vi "Close Device.vi"(8 "error in (no error)":errorcluster, 11 "Device in":refnum<class "Toggle 8.lvclass">) -> (0 "error out":errorcluster, 3 "Device out":refnum<class "Toggle 8.lvclass">)   [LabVIEW 2020, in "Toggle 8.lvclass"]
doc: "Closes the device"
uses:
  Toggle 8.lvclass
  PIC-device/PIC-Device.lvclass
  <instrlib>/Keithley 24XX/Keithley 24XX.lvlib
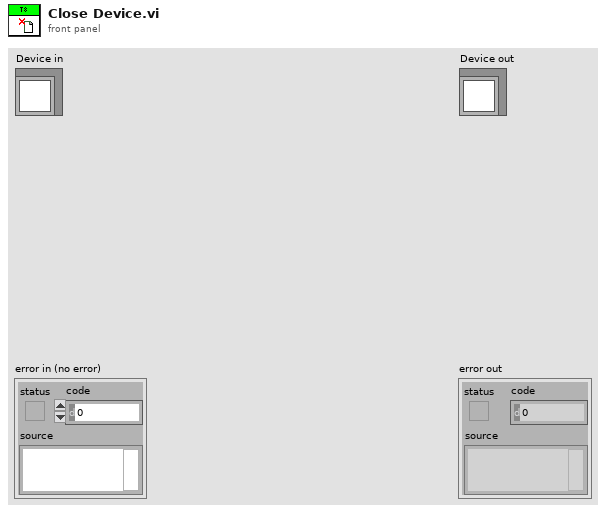
[diagram p1: front panel]
types:
  T1 = cluster{"Enable":bool, "User init values":string}
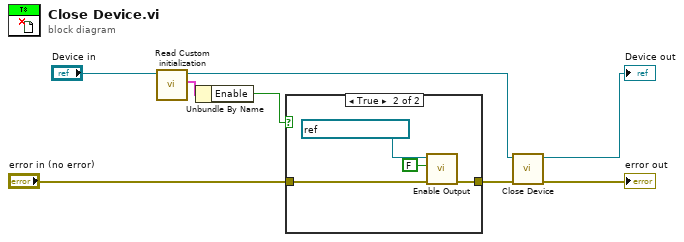
[diagram p0: block diagram]
diagram:
  n1 = call-dynamic "Read Custom initialization.vi"("Toggle 8 in"="Device in") -> ("Custom initialization"=w4:T1, "Toggle 8 out"=w5:refnum<class "Toggle 8.lvclass">)  [unwired: 9 in]
  n2 = Unbundle By Name(w4) -> ("Enable"=w1:bool)
  n3 = case shown="True" w1 {
    tunnel: "error in (no error)" -> [w9 w12]
    tunnel: [w9 w11] -> w2
    frame False {
    }
    frame True {
      n4 = call <instrlib>:"Enable Output.vi"("error in (no error)"=w12, "Enable Output (T: Enable)"=FALSE, "VISA resource name"=refnum<visa-resource-name> "GPIB0::3::INSTR") -> ("error out"=w11:errorcluster)  [unwired: 7 in, 1 out]
    }
  }
  n5 = call-parent "Close Device.vi"("error in (no error)"=w2, "Device in"=w5) -> ("error out"=→"error out":errorcluster, "Device out"=→"Device out":refnum<class "Toggle 8.lvclass">)  [unwired: 8 in]
